vi "lvEtherbone.sdb_find_by_identity.vi"(0 "eb_socket_ID":i32, 1 "eb_device_ID":i32 format="%.0x", 2 "vendor_id":u64 format="%.0x", 3 "device_id":u32 format="%.0x", 5 "error in (no error)":errorcluster) -> (10 "addr_first":u64 format="%.0x", 11 "found?":bool, 12 "addr_last":u64 format="%.0x", 13 "eb_status":T1 items=["EB_SUCCESS"=1, "EB_OK"=0, "EB_FAIL"=-1, "EB_ADDRESS"=-2, "EB_WIDTH"=-3, "EB_OVERFLOW"=-4, "EB_ENDIAN"=-5, "EB_BUSY"=-6, "EB_TIMEOUT"=-7, "EB_OOM"=-8, "EB_ABI"=-9, "EB_SEGFAULT"=-10], 14 "eb_socket_ID out":i32, 15 "eb_device_ID out":i32, 18 "name":string, 19 "error out":errorcluster)   [LabVIEW 2012, in "lvEtherbone.lvlib"]
doc: "/* When scanning by identity, multiple devices may match.\n * The initial value of *devices determines the output space in records.\n * The resulting value of *devices is the number of matching SDB records found.\n * If there are more records than fit in output, they are counted but unwritten.\n * On success, EB_OK is returned. Do not forget to check *devices as well!\n */\nEB_PUBLIC eb_status_t eb_sdb_find_by_identity(eb_device_t device, uint64_t vendor_id, uint32_t device_id, struct sdb_device* output, int* devices);"
uses:
  lvEtherbone.lvlib
  lvEtherbone.lveb_status_t.ctl
  libetherbone.so
panel:
  in  "eb_status_t":T1 items=["EB_SUCCESS"=1, "EB_OK"=0, "EB_FAIL"=-1, "EB_ADDRESS"=-2, "EB_WIDTH"=-3, "EB_OVERFLOW"=-4, "EB_ENDIAN"=-5, "EB_BUSY"=-6, "EB_TIMEOUT"=-7, "EB_OOM"=-8, "EB_ABI"=-9, "EB_SEGFAULT"=-10]
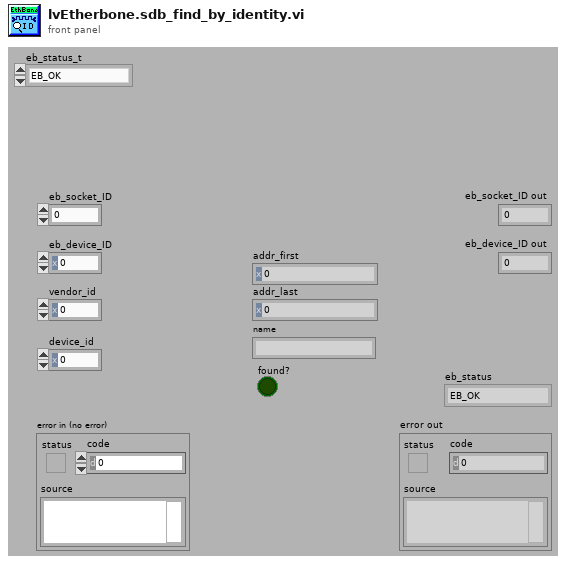
[diagram p1: front panel]
types:
  T1 = typedef "lvEtherbone.lvlib/lvEtherbone.lveb_status_t.ctl" = i32
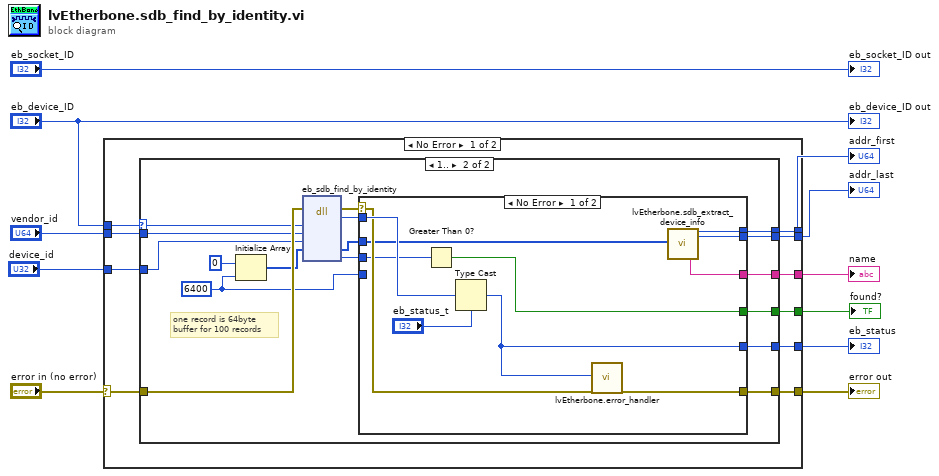
[diagram p0: block diagram]
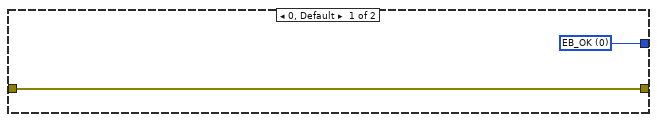
[diagram p2: hidden frame]
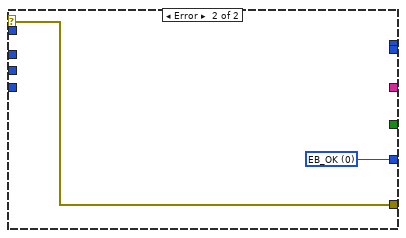
[diagram p3: hidden frame]
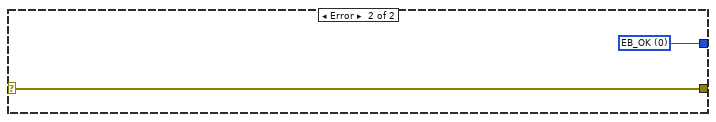
[diagram p4: hidden frame]
diagram:
  n1 = case shown="No Error" "error in (no error)" {
    selector: "error in (no error)" -> [w21 w55]
    tunnel: [w20 w55] -> w10
    tunnel: "vendor_id" -> [w18 _]
    tunnel: "eb_device_ID" -> [w17 _]
    tunnel: [w19 w54] -> w8
    tunnel: [w16 _] -> w5
    tunnel: [w15 _] -> w4
    tunnel: [w14 _] -> w3
    tunnel: "device_id" -> [w13 _]
    tunnel: [w12 _] -> w1
    frame No Error {
      n2 = case shown="1.." w17 {
        selector: w17 -> [_ w33]
        tunnel: w21 -> [w22 w38]
        tunnel: [w22 w37] -> w20
        tunnel: [w23 w36] -> w19
        tunnel: w18 -> [_ w34]
        tunnel: [_ w30] -> w16
        tunnel: [_ w29] -> w15
        tunnel: [_ w28] -> w14
        tunnel: w13 -> [_ w27]
        tunnel: [_ w25] -> w12
        frame 0, Default {
          w23 = T1 0 items=["EB_SUCCESS"=1, "EB_OK"=0, "EB_FAIL"=-1, "EB_ADDRESS"=-2, "EB_WIDTH"=-3, "EB_OVERFLOW"=-4, "EB_ENDIAN"=-5, "EB_BUSY"=-6, "EB_TIMEOUT"=-7, "EB_OOM"=-8, "EB_ABI"=-9, "EB_SEGFAULT"=-10] ("eb_status_t")
        }
        frame 1.. {
          w24 = 6400 ("dimension size")
          # "one record is 64byte\nbuffer for 100 records"
          n3 = Initialize Array(u8 0, w24) -> (w31:u8[])
          n4 = dll-call lib="libetherbone.so" fn="eb_sdb_find_by_identity"(error in=w38, "device"=w33, "vendor_id"=w34, "device_id"=w27, "output"=w31) -> (error out=w39:errorcluster, "eb_status"=w40:i32, "output"=w35:u8[], "devices"=w26:i32)  [unwired: 6 in, 1 out]
          n5 = case shown="No Error" w39 {
            selector: w39 -> [w48 w53]
            tunnel: w40 -> [w51 _]
            tunnel: [w49 w52] -> w36
            tunnel: [w47 w53] -> w37
            tunnel: w35 -> [w41 _]
            tunnel: [w46 _] -> w30
            tunnel: [w45 _] -> w29
            tunnel: [w44 _] -> w28
            tunnel: w26 -> [w43 _]
            tunnel: [w42 _] -> w25
            tunnel: w24 -> [_ _]
            frame No Error {
              n6 = Greater Than 0?(x=w43) -> (x > 0?=w42:bool)
              n7 = Type Cast(type="eb_status_t", x=w51) -> (*(type *) &x=w49:T1)
              n8 = call "lvEtherbone.error_handler.vi"("eb_status"=w49, "error in"=w48) -> ("error out"=w47:errorcluster)  [unwired: 17 in]
              n9 = call "lvEtherbone.sdb_extract_device_info.vi"("sdb_device_bin"=w41) -> ("name"=w44:string, "addr_first"=w46:u64, "addr_last"=w45:u64)  [unwired: 11 in, 5 out]
            }
            frame Error {
              w52 = T1 0 items=["EB_SUCCESS"=1, "EB_OK"=0, "EB_FAIL"=-1, "EB_ADDRESS"=-2, "EB_WIDTH"=-3, "EB_OVERFLOW"=-4, "EB_ENDIAN"=-5, "EB_BUSY"=-6, "EB_TIMEOUT"=-7, "EB_OOM"=-8, "EB_ABI"=-9, "EB_SEGFAULT"=-10] ("eb_status_t")
            }
          }
        }
      }
    }
    frame Error {
      w54 = T1 0 items=["EB_SUCCESS"=1, "EB_OK"=0, "EB_FAIL"=-1, "EB_ADDRESS"=-2, "EB_WIDTH"=-3, "EB_OVERFLOW"=-4, "EB_ENDIAN"=-5, "EB_BUSY"=-6, "EB_TIMEOUT"=-7, "EB_OOM"=-8, "EB_ABI"=-9, "EB_SEGFAULT"=-10] ("eb_status_t")
    }
  }
  "error out" <- w10
  "eb_status" <- w8
  "addr_first" <- w5
  "addr_last" <- w4
  "name" <- w3
  "found?" <- w1
  "eb_socket_ID out" <- "eb_socket_ID"
  "eb_device_ID out" <- "eb_device_ID"
